vi "T7-FullModbus.vi"(6 "MaxAge(s)":dbl, 9 "Value to Output":dbl, 10 "Ch Description":T2 {"Duty" format="%016b"; "D" format="%#_5g"; "C" format="%#_5g"; "B" format="%#_5g"; "A" format="%#_5g"}) -> (2 "Output Value":dbl, 3 "String":string)   [LabVIEW 2020]
uses:
  ADAM Client/Sub VIs/ADAM Controls/Ch_description_ADAM.ctl
  ADAM Client/Sub VIs/ADAM Controls/Module_type_ADAM.ctl
  ADAM Client/Sub VIs/ADAM Controls/Function_ADAM.ctl
  ADAM Client/Sub VIs/ADAM Controls/Channel_State.ctl
  ADAM Client/Sub VIs/ADAM Controls/Calib_type_ADAM.ctl
  ADAM Client/Sub VIs/ADAM Controls/Address.ctl
  Serial Link Layer/Modbus/RegisterTypes.ctl
  ADAM Client/Sub VIs/ADAM Controls/Remember_value_mode.ctl
  <vilib>/Utility/error.llb/DialogType.ctl
panel:
  in  "ValidRegisterTypes":T1
  out "ValidDataTypes":string[](array[string])=["BYTE", "UINT16", "UINT32", "UINT64", "INT32", "FLOAT32", "STRING", "ADAM32"]
  # "The Red (Comments) box should be used to indicate the data type, optionally followed by :RegisterType."
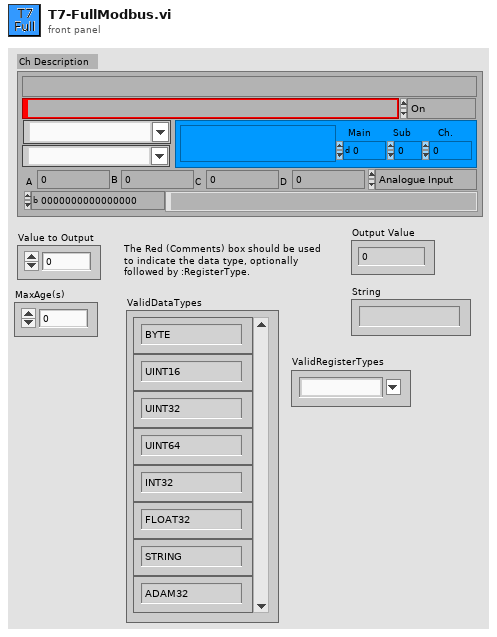
[diagram p1: front panel]
types:
  T1 = typedef "RegisterTypes.ctl" = string
  T2 = typedef "Ch_description_ADAM.ctl" = cluster{"Ch Name":string, "Type":T3, "Function":T4, "Ch State":T5, "Calibration type":T6, "A":dbl, "B":dbl, "C":dbl, "D":dbl, "Comments":string, "Address":T7, "String":string, "Duty":u16}
  T3 = typedef "Module_type_ADAM.ctl" = string
  T4 = typedef "Function_ADAM.ctl" = enum16{"Analogue Input", "Digital Input", "Event counter", "Event rate", "Analogue Output", "Digital Output", "Relay Output"}
  T5 = typedef "Channel_State.ctl" = enum16{"On", "Off", "Always On", "Always Off"}
  T6 = typedef "Calib_type_ADAM.ctl" = string
  T7 = typedef "Address.ctl" = cluster{"Main":i32, "Ch.":i32, "Sub":i32, "Port Name":string}
  T8 = typedef "Remember_value_mode.ctl" = enum16{"Read only", "Read and Write"}
  T9 = typedef "DialogType.ctl" = u16
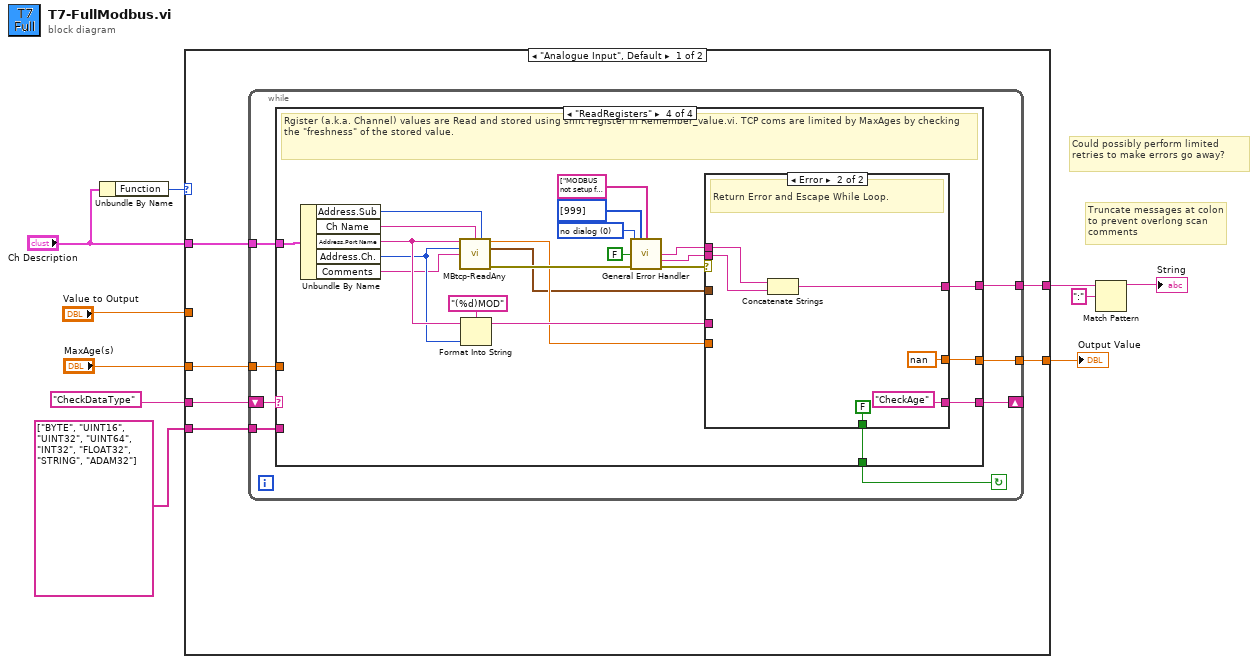
[diagram p0: block diagram]
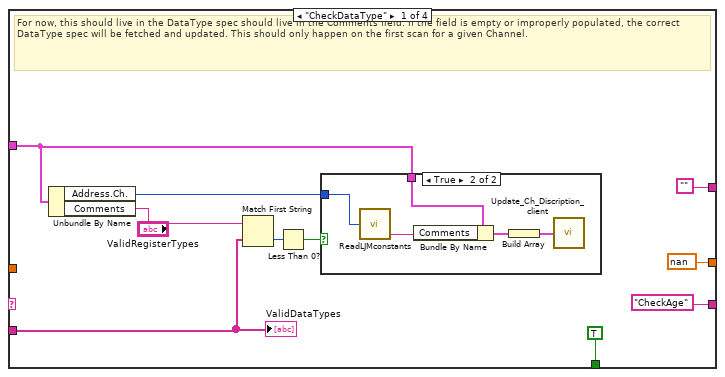
[diagram p2: hidden frame]
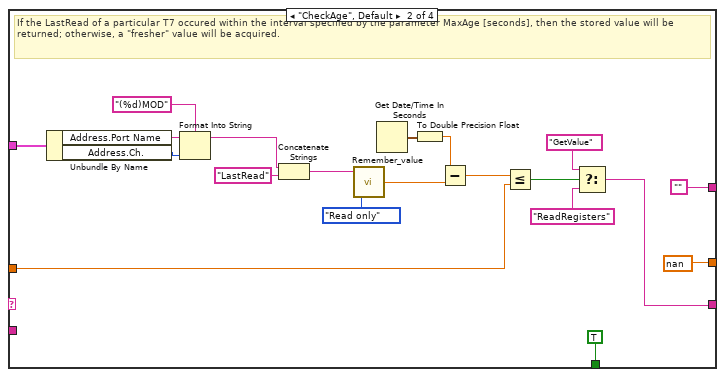
[diagram p4: hidden frame]
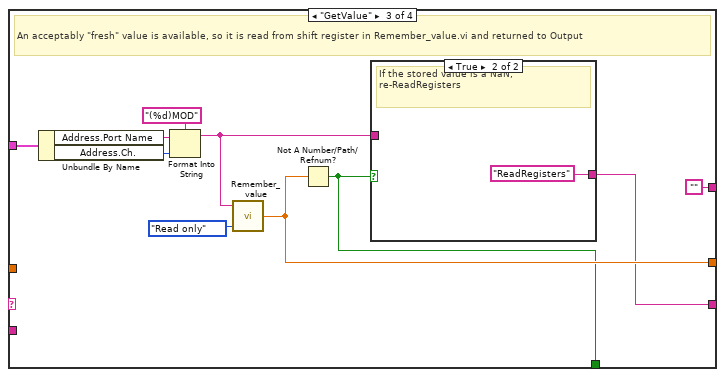
[diagram p5: hidden frame]
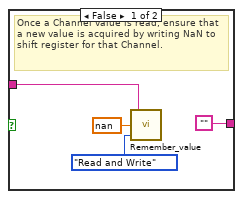
[diagram p6: hidden frame]
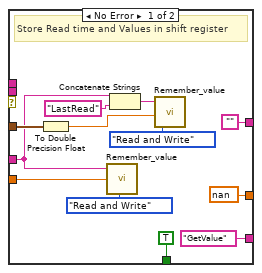
[diagram p7: hidden frame]
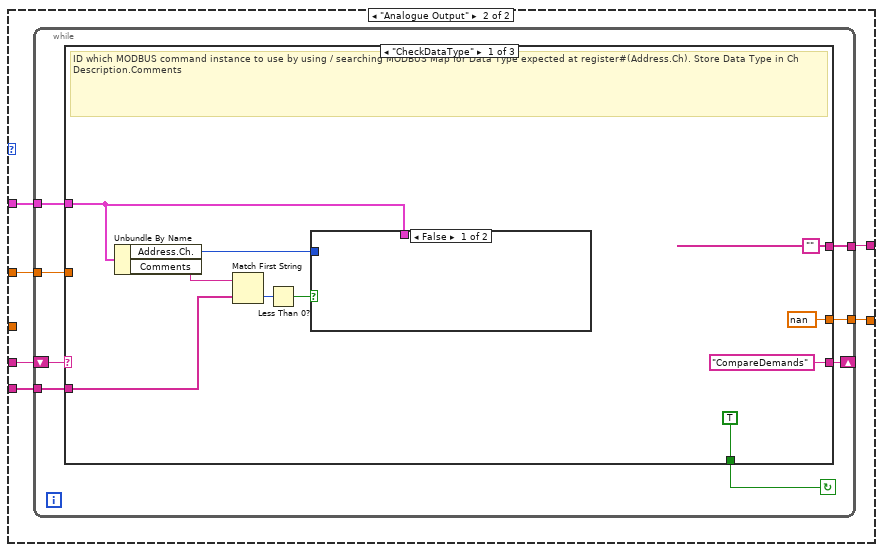
[diagram p8: hidden frame]
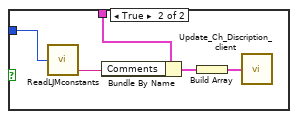
[diagram p9: hidden frame]
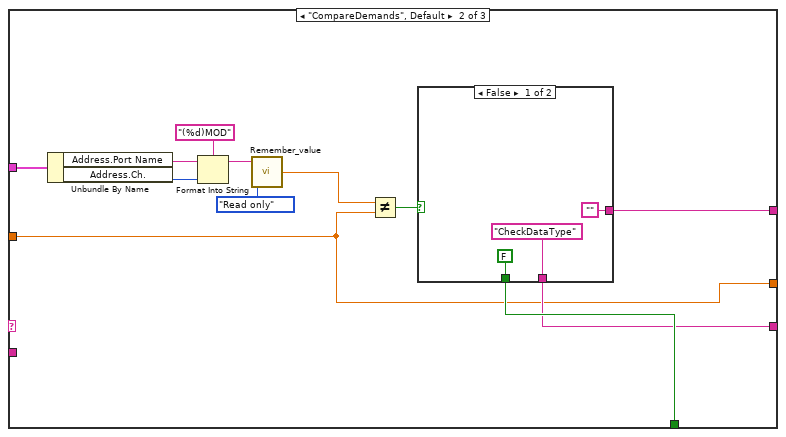
[diagram p10: hidden frame]
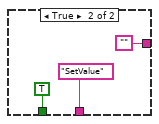
[diagram p11: hidden frame]
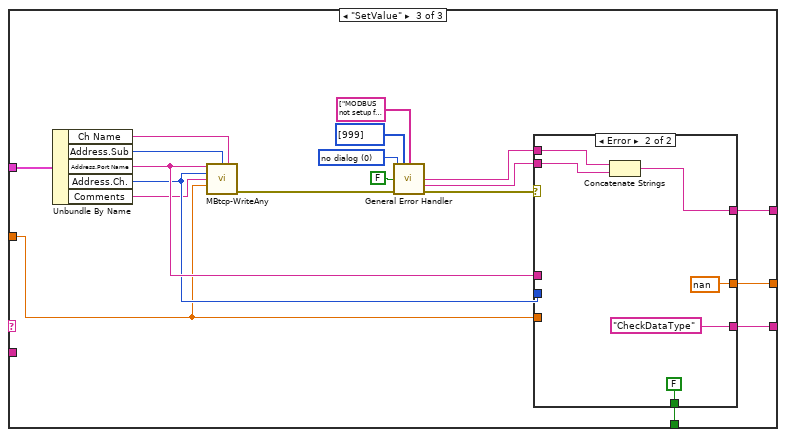
[diagram p12: hidden frame]
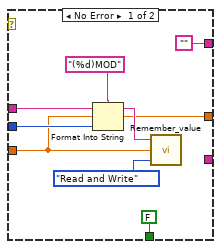
[diagram p13: hidden frame]
diagram:
  # "Could possibly perform limited retries to make errors go away?"
  # "Truncate messages at colon to prevent overlong scan comments"
  n1 = Unbundle By Name("Ch Description") -> ("Function"=w6:T4)
  n2 = case shown="\"Analogue Input\", Default" w6 {
    tunnel: "Ch Description" -> [w16 w120]
    tunnel: [w15 w118] -> w2
    tunnel: [w14 w117] -> w9
    tunnel: "Value to Output" -> [_ w119]
    tunnel: "MaxAge(s)" -> [w13 _]
    tunnel: "CheckDataType" -> [w12 w116]
    tunnel: string[] ["BYTE", "UINT16", "UINT32", "UINT64", "INT32", "FLOAT32", "STRING", "ADAM32"] ("Array") -> [w11 w115]
    frame "Analogue Input", Default {
      n3 = while {
        shift-right: [w19] -> _
        shift-left: w12 -> [w24]
        tunnel: w16 -> [w23]
        tunnel: [w20] -> w15
        tunnel: [w21] -> w14
        tunnel: w13 -> [w18]
        tunnel: w11 -> [w17]
        stop <- w22 continue-if-true
        n4 = case shown="\"ReadRegisters\"" w24 {
          tunnel: ["" "" "" w95] -> w20
          tunnel: ["CheckAge" w49 w66 w94] -> w19
          tunnel: [TRUE TRUE w65 w93] -> w22
          tunnel: [nan ("Output Value") nan w67 w92] -> w21
          tunnel: w23 -> [w30 w45 w63 w91]
          tunnel: w18 -> [_ w40 _ _]
          tunnel: w17 -> [w25 _ _ _]
          frame "CheckDataType" {
            # "For now, this should live in the DataType spec should live in the Comments field. If the field is empty or improperly populated, the correct DataType spec will be fetched and updated. This should only happen on the first scan for a given Channel."
            n5 = Unbundle By Name(w30) -> ("Address.Ch."=w34:i32, "Comments"=w31:string)
            n6 = Match First String(2:w25, 3:w31) -> (0:w32:i32)  [unwired: 1 out]
            n7 = Less Than 0?(x=w32) -> (x < 0?=w33:bool)
            n8 = case shown="True" w33 {
              tunnel: w34 -> [_ w39]
              tunnel: w30 -> [_ w36]
              frame False {
              }
              frame True {
                n9 = call "ReadLJMconstants.vi"("Selected Register"=w39) -> ("Data Type"=w35:string)  [unwired: 2 out]
                n10 = Bundle By Name(cluster=w36, "Comments"=w35) -> (w37:T2)
                n11 = Build Array(w37) -> (w38:T2[])
                n12 = call "Update_Ch_Discription_client.vi"("Channels to update In"=w38) -> ()  [unwired: 1 out]
              }
            }
            "ValidDataTypes" <- w25
          }
          frame "CheckAge", Default {
            # "If the LastRead of a particular T7 occured within the interval specified by the parameter MaxAge [seconds], then the stored value will be returned; otherwise, a \"fresher\" value will be acquired."
            n13 = Unbundle By Name(w45) -> ("Address.Port Name"=w43:string, "Address.Ch."=w42:i32)
            n14 = Format Into String(format string="(%d)MOD", initial string=w43, w42) -> (resulting string=w41:string)  [unwired: 1 in, 1 out]
            n15 = Concatenate Strings(w41, "LastRead" ("string")) -> (w59:string)
            n16 = call "Remember_value.vi"("Mode"=Remember_value_mode."Read only", "Ch name"=w59) -> ("Output Value"=w54:dbl)  [unwired: 1 in]
            n17 = Get Date/Time In Seconds() -> (seconds since 1Jan1904=w56:timestamp)
            n18 = To Double Precision Float(number=w56) -> (double precision float=w55:dbl)
            n19 = Subtract(x=w55, y=w54) -> (x-y=w53:dbl)
            n20 = Less Or Equal?(x=w53, y=w40) -> (x <= y?=w52:bool)
            n21 = Select(t="GetValue", s=w52, f="ReadRegisters") -> (s? t:f=w49:string)
          }
          frame "GetValue" {
            # "An acceptably \"fresh\" value is available, so it is read from shift register in Remember_value.vi and returned to Output"
            n22 = Unbundle By Name(w63) -> ("Address.Port Name"=w61:string, "Address.Ch."=w60:i32)
            n23 = Format Into String(format string="(%d)MOD", initial string=w61, w60) -> (resulting string=w64:string)  [unwired: 1 in, 1 out]
            n24 = call "Remember_value.vi"("Mode"=Remember_value_mode."Read only", "Ch name"=w64) -> ("Output Value"=w67:dbl)  [unwired: 1 in]
            n25 = Not A Number/Path/Refnum?(number/path/refnum=w67) -> (NaN/Path/Refnum?=w65:bool)
            n26 = case shown="True" w65 {
              tunnel: ["" "ReadRegisters"] -> w66
              tunnel: w64 -> [w72 _]
              frame False {
                # "Once a Channel value is read, ensure that a new value is acquired by writing NaN to shift register for that Channel."
                n27 = call "Remember_value.vi"("Mode"=Remember_value_mode."Read and Write", "Input Value"=nan, "Ch name"=w72) -> ()  [unwired: 1 out]
              }
              frame True {
                # "If the stored value is a NaN, re-ReadRegisters"
              }
            }
          }
          frame "ReadRegisters" {
            w96 = T9 0 items=["no dialog", "OK message", "continue or stop message", "OK message + warnings", "continue/stop + warnings"] ("type of dialog (OK msg:1)")
            # "Rgister (a.k.a. Channel) values are Read and stored using shift register in Remember_value.vi. TCP coms are limited by MaxAges by checking the \"freshness\" of the stored value."
            n28 = Unbundle By Name(w91) -> ("Address.Sub"=w76:i32, "Ch Name"=w84:string, "Address.Port Name"=w83:string, "Address.Ch."=w82:i32, "Comments"=w75:string)
            n29 = call "MBtcp-ReadAny.vi"("IP Address"=w83, "Ch Name"=w84, "Slave ID"=w76, "Register"=w82, "DataType(:RegisterType)"=w75) -> ("Value"=w80:dbl, "Read At"=w79:timestamp, "error out"=w88:errorcluster)  [unwired: 8 in]
            n30 = Format Into String(format string="(%d)MOD", initial string=w83, w82) -> (resulting string=w89:string)  [unwired: 1 in, 1 out]
            n31 = call <vilib>:"General Error Handler.vi"("[user-defined codes]"=i32[] [999], "[user-defined descriptions]"=string[] ["MODBUS not setup for DataType"], "search ni.com link visible?(T)"=FALSE, "type of dialog (OK msg:1)"=w96, "error in (no error)"=w88) -> ("source out"=w78:string, "message"=w77:string, "error out"=w81:errorcluster)  [unwired: 6 in, 2 out]
            n32 = case shown="Error" w81 {
              tunnel: w77 -> [_ w113]
              tunnel: w78 -> [_ w114]
              tunnel: ["" w109] -> w95
              tunnel: w80 -> [w104 _]
              tunnel: w79 -> [w103 _]
              tunnel: ["GetValue" "CheckAge"] -> w94
              tunnel: [TRUE FALSE] -> w93
              tunnel: [nan nan] -> w92
              tunnel: w89 -> [w97 _]
              frame No Error {
                # "Store Read time and Values in shift register"
                n33 = To Double Precision Float(number=w103) -> (double precision float=w102:dbl)
                n34 = call "Remember_value.vi"("Mode"=Remember_value_mode."Read and Write", "Input Value"=w104, "Ch name"=w97) -> ()  [unwired: 1 out]
                n35 = Concatenate Strings(w97, "LastRead" ("string")) -> (w107:string)
                n36 = call "Remember_value.vi"("Mode"=Remember_value_mode."Read and Write", "Input Value"=w102, "Ch name"=w107) -> ()  [unwired: 1 out]
              }
              frame Error {
                # "Return Error and Escape While Loop."
                n37 = Concatenate Strings(w114, w113) -> (w109:string)
              }
            }
          }
        }
      }
    }
    frame "Analogue Output" {
      n38 = while {
        tunnel: w120 -> [w128]
        tunnel: [w126] -> w118
        tunnel: w119 -> [w127]
        tunnel: [w125] -> w117
        shift-right: [w124] -> _
        shift-left: w116 -> [w122]
        tunnel: w115 -> [w121]
        stop <- w123 continue-if-true
        n39 = case shown="\"CheckDataType\"" w122 {
          tunnel: w128 -> [w131 w152 w171]
          tunnel: w127 -> [_ w144 w162]
          tunnel: ["" w145 w180] -> w126
          tunnel: [nan ("Output Value") w144 w179] -> w125
          tunnel: ["CompareDemands" w146 w178] -> w124
          tunnel: [TRUE w147 w177] -> w123
          tunnel: w121 -> [w129 _ _]
          frame "CheckDataType" {
            # "ID which MODBUS command instance to use by using / searching MODBUS Map for Data Type expected at register#(Address.Ch). Store Data Type in Ch Description.Comments"
            n40 = Unbundle By Name(w131) -> ("Address.Ch."=w138:i32, "Comments"=w135:string)
            n41 = Match First String(2:w129, 3:w135) -> (0:w136:i32)  [unwired: 1 out]
            n42 = Less Than 0?(x=w136) -> (x < 0?=w137:bool)
            n43 = case shown="False" w137 {
              tunnel: w138 -> [_ w143]
              tunnel: w131 -> [_ w140]
              frame False {
              }
              frame True {
                n44 = call "ReadLJMconstants.vi"("Selected Register"=w143) -> ("Data Type"=w139:string)  [unwired: 2 out]
                n45 = Bundle By Name(cluster=w140, "Comments"=w139) -> (w141:T2)
                n46 = Build Array(w141) -> (w142:T2[])
                n47 = call "Update_Ch_Discription_client.vi"("Channels to update In"=w142) -> ()  [unwired: 1 out]
              }
            }
          }
          frame "CompareDemands", Default {
            n48 = Unbundle By Name(w152) -> ("Address.Port Name"=w151:string, "Address.Ch."=w150:i32)
            n49 = Format Into String(format string="(%d)MOD", initial string=w151, w150) -> (resulting string=w155:string)  [unwired: 1 in, 1 out]
            n50 = call "Remember_value.vi"("Mode"=Remember_value_mode."Read only", "Ch name"=w155) -> ("Output Value"=w149:dbl)  [unwired: 1 in]
            n51 = Not Equal?(x=w149, y=w144) -> (x != y?=w148:bool)
            n52 = case shown="False" w148 {
              tunnel: [FALSE TRUE] -> w147
              tunnel: ["CheckDataType" "SetValue"] -> w146
              tunnel: ["" ""] -> w145
              frame False {
              }
              frame True {
              }
            }
          }
          frame "SetValue" {
            w176 = T9 0 items=["no dialog", "OK message", "continue or stop message", "OK message + warnings", "continue/stop + warnings"] ("type of dialog (OK msg:1)")
            n53 = Unbundle By Name(w171) -> ("Ch Name"=w167:string, "Address.Sub"=w164:i32, "Address.Port Name"=w166:string, "Address.Ch."=w165:i32, "Comments"=w163:string)
            n54 = call "MBtcp-WriteAny.vi"("IP Address"=w166, "Slave ID"=w164, "Ch Name"=w167, "Register"=w165, "DataType(:RegisterType)"=w163, "Value to Output"=w162) -> ("error out"=w175:errorcluster)  [unwired: 9 in]
            n55 = call <vilib>:"General Error Handler.vi"("[user-defined codes]"=i32[] [999], "[user-defined descriptions]"=string[] ["MODBUS not setup for DataType"], "search ni.com link visible?(T)"=FALSE, "type of dialog (OK msg:1)"=w176, "error in (no error)"=w175) -> ("source out"=w169:string, "message"=w168:string, "error out"=w170:errorcluster)  [unwired: 6 in, 2 out]
            n56 = case shown="Error" w170 {
              tunnel: w169 -> [_ w194]
              tunnel: w168 -> [_ w193]
              tunnel: ["" w192] -> w180
              tunnel: [w181 nan ("Output Value")] -> w179
              tunnel: w166 -> [w184 _]
              tunnel: [_ "CheckDataType"] -> w178
              tunnel: [FALSE FALSE] -> w177
              tunnel: w165 -> [w182 _]
              tunnel: w162 -> [w181 _]
              frame No Error {
                n57 = Format Into String(format string="(%d)MOD", initial string=w184, w182) -> (resulting string=w187:string)  [unwired: 1 in, 1 out]
                n58 = call "Remember_value.vi"("Mode"=Remember_value_mode."Read and Write", "Input Value"=w181, "Ch name"=w187) -> ()  [unwired: 1 out]
              }
              frame Error {
                n59 = Concatenate Strings(w194, w193) -> (w192:string)
              }
            }
          }
        }
      }
    }
  }
  "Output Value" <- w9
  n60 = Match Pattern(string=w2, regular expression=":") -> (before substring=→"String":string)  [unwired: 1 in, 3 out]
